vi "Scope_FPGA_v00.vi"(0 "Scope IPs":T3, 9 "Scope":T1, 11 "Lock Select":T4, 12 "Cavities Data":u64[](array[numeric]), 13 "XY HD ON":bool, 14 "Graph Data":u64[](array[numeric])) -> (1 "xy HD A":cluster{i16[], i16[]}(graph), 2 "xy HD B":cluster{i16[], i16[]}(graph), 3 "Scope OP Graph":cluster{dbl[], dbl[]}[](graph), 4 "Scope Cavities ON":bool, 6 "Scope Graph ON":bool, 8 "error":dbl[](array[numeric]), 10 "Scope Cavities":T2, 15 "Scope Graph":T2)   [LabVIEW 2010]
doc: "Creates an oscilliscope graph from the FIFO data, as well as packages data structures for FPGA_Cavities via the reference."
uses:
  Strict Type Defs/Lock Select.ctl
  Strict Type Defs/Lock or Hold.ctl
panel:
  out "Scope OPs (for saving)":cluster{dbl[], i16[], i16[], i16[], i16[]}
  in  "Scope":T2={"Trigger Direction"=enum."minus-plus", "Delay"=0, "Aquisition Rate (Ticks)"=20, "Offset"=0, "Channel"=0, "Channel Selector"={"Channel 1"=0, "Channel 2"=0, "Channel 3"=0, "Channel 4"=0}}
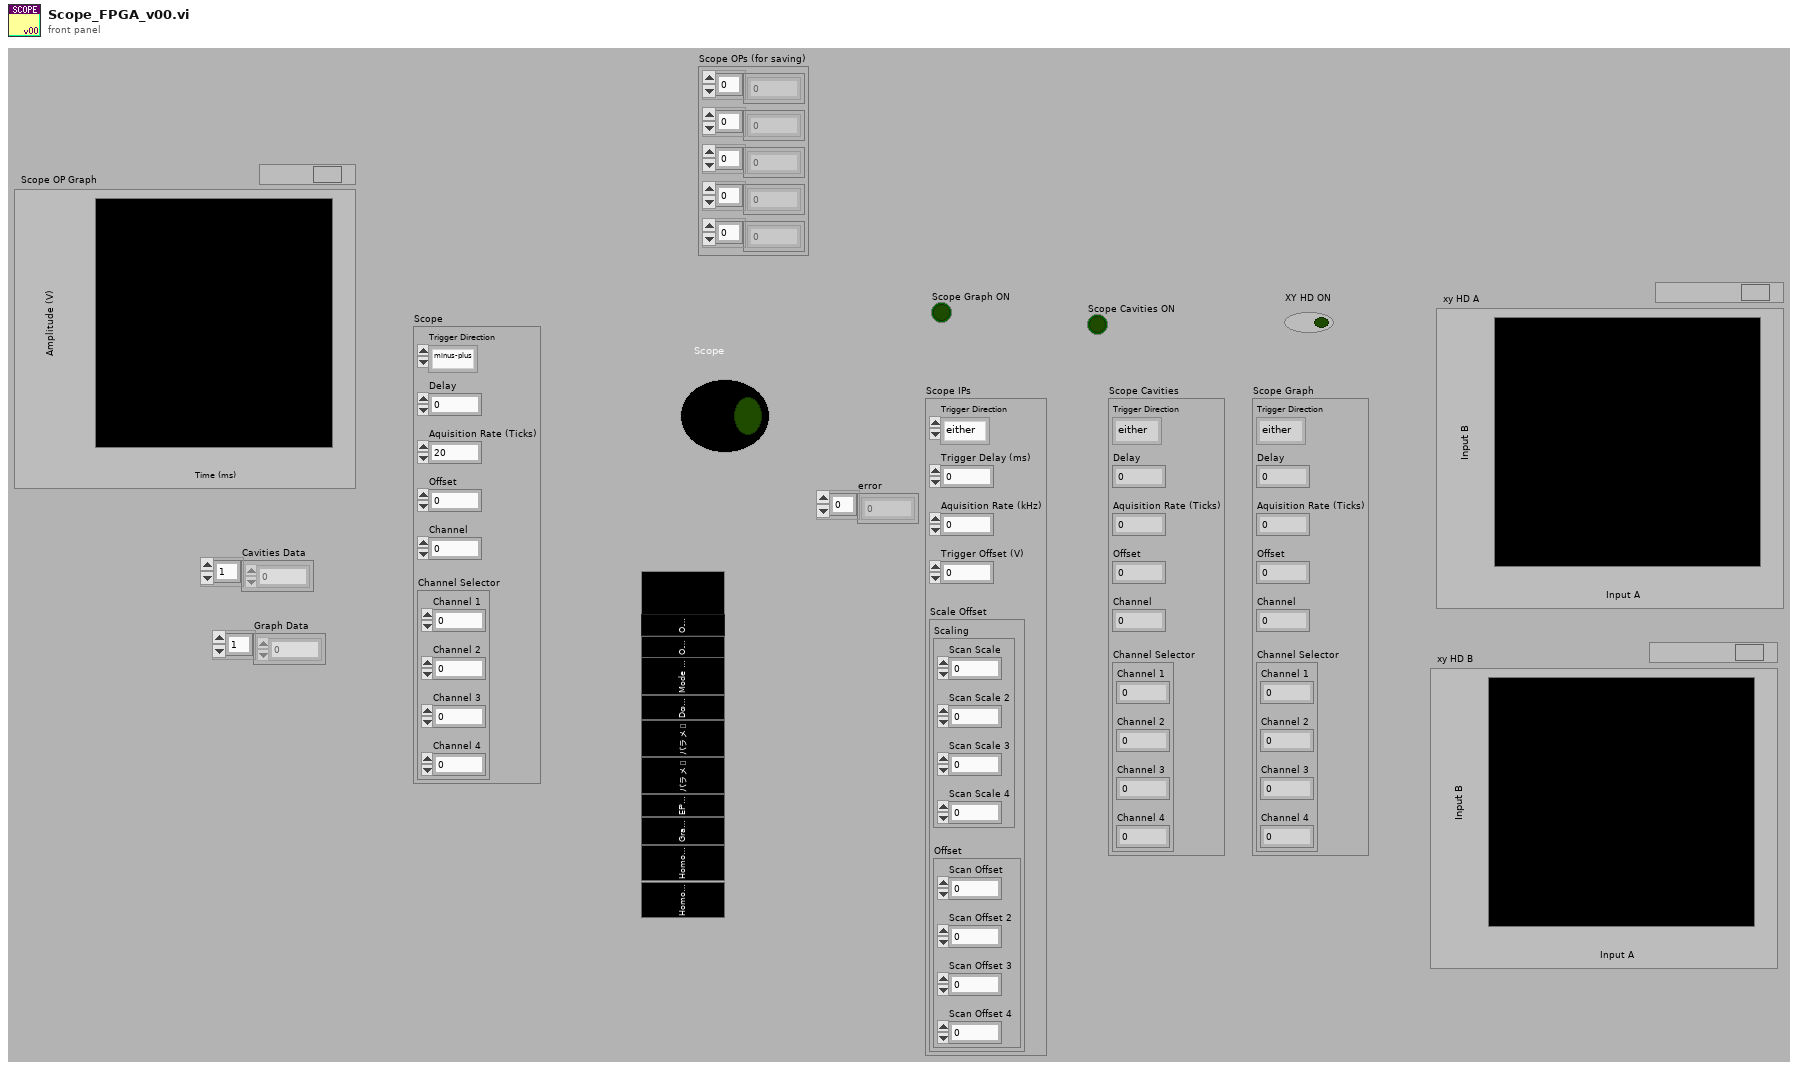
[diagram p1: front panel]
types:
  T1 = typedef "Lock or Hold.ctl" = bool
  T2 = cluster{"Trigger Direction":enum8{"either", "minus-plus", "plus-minus"}, "Delay":u32, "Aquisition Rate (Ticks)":u32, "Offset":i16, "Channel":i32, "Channel Selector":cluster{"Channel 1":i32, "Channel 2":i32, "Channel 3":i32, "Channel 4":i32}}
  T3 = cluster{"Trigger Direction":enum8{"either", "minus-plus", "plus-minus"}, "Trigger Delay (ms)":dbl, "Aquisition Rate (kHz)":dbl, "Trigger Offset (V)":dbl, "Scale Offset":cluster{"Scaling":cluster{"Scan Scale":i16, "Scan Scale 2":i16, "Scan Scale 3":i16, "Scan Scale 4":i16}, "Offset":cluster{"Scan Offset":i16, "Scan Offset 2":i16, "Scan Offset 3":i16, "Scan Offset 4":i16}}}
  T4 = typedef "Lock Select.ctl" = enum32{"OPO A", "OPO B", "Mode Cleaner", "Doubler", "パラメ OPO A", "パラメ OPO B", "EPR BS", "Graph BS", "Homodyne A", "Homodyne B"}
  T5 = cluster{"Channel 1":i32, "Channel 2":i32, "Channel 3":i32, "Channel 4":i32}
  T6 = cluster{"Scan Offset":i16, "Scan Offset 2":i16, "Scan Offset 3":i16, "Scan Offset 4":i16}
  T7 = cluster{"Scan Scale":i16, "Scan Scale 2":i16, "Scan Scale 3":i16, "Scan Scale 4":i16}
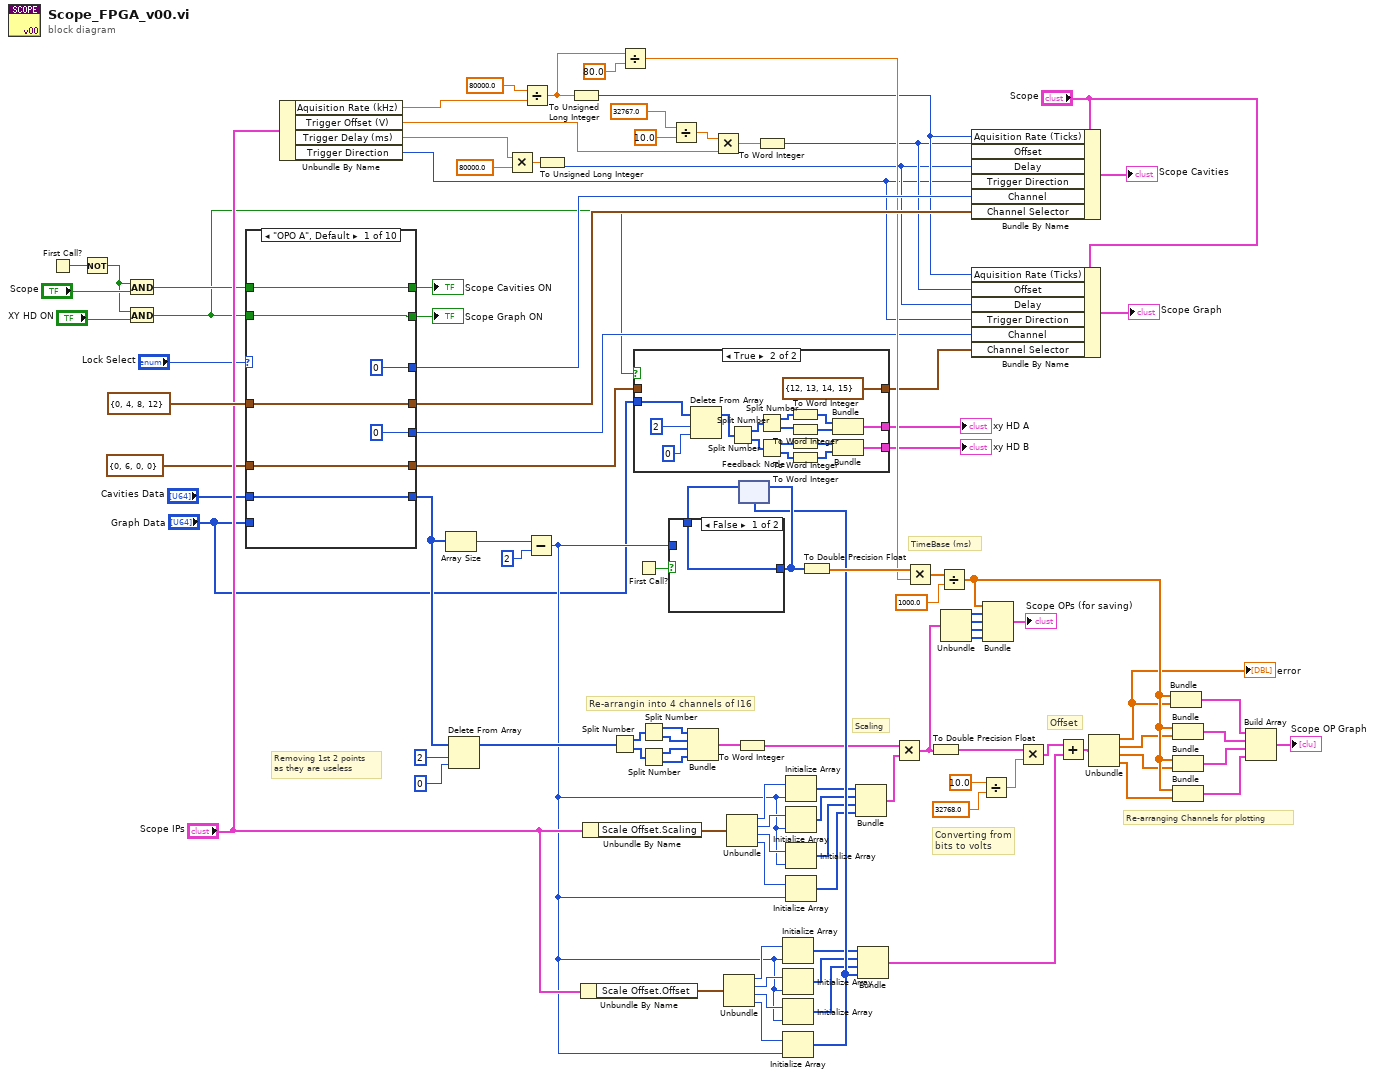
[diagram p0: block diagram]
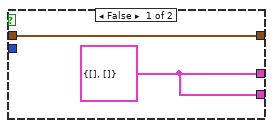
[diagram p2: hidden frame]
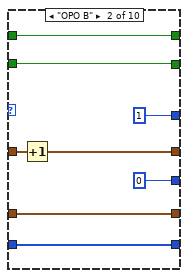
[diagram p4: hidden frame]
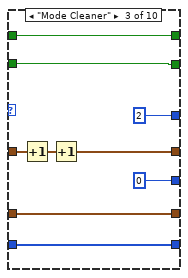
[diagram p5: hidden frame]
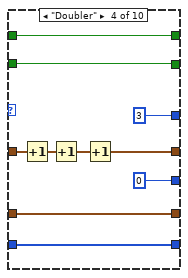
[diagram p6: hidden frame]
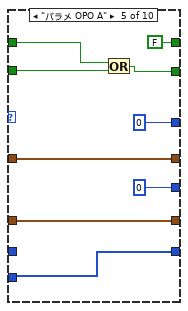
[diagram p7: hidden frame]
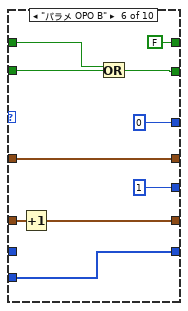
[diagram p8: hidden frame]
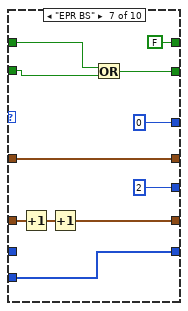
[diagram p9: hidden frame]
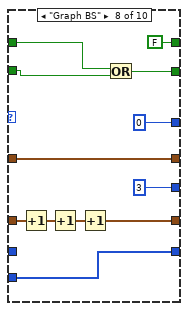
[diagram p10: hidden frame]
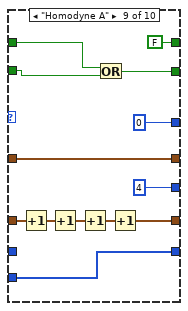
[diagram p11: hidden frame]
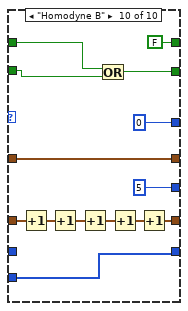
[diagram p12: hidden frame]
diagram:
  # "TimeBase (ms)"
  # "Re-arranging Channels for plotting"
  # "Re-arrangin into 4 channels of I16"
  # "Converting from\nbits to volts"
  # "Offset"
  # "Scaling"
  # "Removing 1st 2 points\nas they are useless"
  n1 = First Call?() -> (First Call?: T/F=w15:bool)
  n2 = Not(x=w15) -> (.not. x?=w7:bool)
  n3 = And(x=w7, y="Scope") -> (x .and. y?=w13:T1)
  n4 = And(x=w7, y="XY HD ON") -> (x .and. y?=w4:bool)
  n5 = case shown="\"OPO A\", Default" "Lock Select" {
    tunnel: T5 {"Channel 1"=0, "Channel 2"=4, "Channel 3"=8, "Channel 4"=12} ("Channel Selector") -> [w111 w116 w125 w135 w145 w155 w166 w178 w191 w205]
    tunnel: [w111 w115 w123 w131 w145 w155 w166 w178 w191 w205] -> w94
    tunnel: [0 1 2 3 0 0 0 0 0 0] -> w93
    tunnel: [w110 w119 w128 w138 w143 w152 w162 w173 w185 w198] -> w25
    tunnel: "Cavities Data" -> [w110 w119 w128 w138 _ _ _ _ _ _]
    tunnel: "Graph Data" -> [_ _ _ _ w143 w152 w162 w173 w185 w198]
    tunnel: [0 ("Channel") 0 ("Channel") 0 ("Channel") 0 ("Channel") 0 ("Channel") 1 ("Channel") 2 ("Channel") 3 ("Channel") 4 ("Channel") 5 ("Channel")] -> w17
    tunnel: T5 {"Channel 1"=0, "Channel 2"=6, "Channel 3"=0, "Channel 4"=0} ("Channel Selector") -> [w107 w114 w122 w133 w144 w154 w165 w177 w190 w204]
    tunnel: [w107 w114 w122 w133 w144 w153 w163 w174 w186 w199] -> w6
    tunnel: [w106 w113 w121 w130 T1 FALSE ("Scope") T1 FALSE ("Scope") T1 FALSE ("Scope") T1 FALSE ("Scope") T1 FALSE ("Scope") T1 FALSE ("Scope")] -> w14
    tunnel: w13 -> [w106 w113 w121 w130 w140 w148 w158 w169 w181 w194]
    tunnel: [w105 w112 w120 w129 w139 w149 w160 w171 w183 w196] -> w11
    tunnel: w4 -> [w105 w112 w120 w129 w141 w150 w159 w170 w182 w195]
    frame "OPO A", Default {
    }
    frame "OPO B" {
      n6 = Increment(x=w116) -> (x+1=w115:T5)
    }
    frame "Mode Cleaner" {
      n7 = Increment(x=w125) -> (x+1=w124:T5)
      n8 = Increment(x=w124) -> (x+1=w123:T5)
    }
    frame "Doubler" {
      n9 = Increment(x=w135) -> (x+1=w134:T5)
      n10 = Increment(x=w134) -> (x+1=w132:T5)
      n11 = Increment(x=w132) -> (x+1=w131:T5)
    }
    frame "パラメ OPO A" {
      n12 = Or(x=w140, y=w141) -> (x .or. y?=w139:T1)
    }
    frame "パラメ OPO B" {
      n13 = Increment(x=w154) -> (x+1=w153:T5)
      n14 = Or(x=w148, y=w150) -> (x .or. y?=w149:T1)
    }
    frame "EPR BS" {
      n15 = Increment(x=w165) -> (x+1=w164:T5)
      n16 = Increment(x=w164) -> (x+1=w163:T5)
      n17 = Or(x=w158, y=w159) -> (x .or. y?=w160:T1)
    }
    frame "Graph BS" {
      n18 = Increment(x=w177) -> (x+1=w176:T5)
      n19 = Increment(x=w176) -> (x+1=w175:T5)
      n20 = Increment(x=w175) -> (x+1=w174:T5)
      n21 = Or(x=w169, y=w170) -> (x .or. y?=w171:T1)
    }
    frame "Homodyne A" {
      n22 = Increment(x=w190) -> (x+1=w189:T5)
      n23 = Increment(x=w189) -> (x+1=w188:T5)
      n24 = Increment(x=w188) -> (x+1=w187:T5)
      n25 = Or(x=w181, y=w182) -> (x .or. y?=w183:T1)
      n26 = Increment(x=w187) -> (x+1=w186:T5)
    }
    frame "Homodyne B" {
      n27 = Increment(x=w204) -> (x+1=w203:T5)
      n28 = Increment(x=w203) -> (x+1=w202:T5)
      n29 = Increment(x=w202) -> (x+1=w201:T5)
      n30 = Or(x=w194, y=w195) -> (x .or. y?=w196:T1)
      n31 = Increment(x=w201) -> (x+1=w200:T5)
      n32 = Increment(x=w200) -> (x+1=w199:T5)
    }
  }
  "Scope Cavities ON" <- w14
  "Scope Graph ON" <- w11
  n33 = Unbundle By Name("Scope IPs") -> ("Aquisition Rate (kHz)"=w103:dbl, "Trigger Offset (V)"=w98:dbl, "Trigger Delay (ms)"=w96:dbl, "Trigger Direction"=w18:enum8{"either", "minus-plus", "plus-minus"})
  n34 = Array Size(array=w25) -> (size(s)=w87:i32)
  n35 = Delete From Array(array=w25, length=2, index=0) -> (array with subset deleted=w32:u64[])  [unwired: 1 out]
  n36 = Multiply(x=w96, y=80000.0) -> (x*y=w97:dbl)
  n37 = Divide(x=80000.0, y=w103) -> (x/y=w91:dbl)
  n38 = Subtract(x=w87, y=2) -> (x-y=w10:i32)
  n39 = To Unsigned Long Integer(number=w97) -> (unsigned 32bit integer=w19:u32)
  n40 = To Unsigned Long Integer(number=w91) -> (unsigned 32bit integer=w21:u32)
  n41 = Unbundle By Name("Scope IPs") -> ("Scale Offset.Offset"=w41:T6)
  n42 = Unbundle By Name("Scope IPs") -> ("Scale Offset.Scaling"=w57:T7)
  n43 = Split Number(x=w32) -> (hi(x)=w34:u32[], lo(x)=w33:u32[])
  n44 = Divide(x=w91, y=80.0) -> (x/y=w31:dbl)
  n45 = case shown="True" w4 {
    tunnel: w6 -> [w209 _]
    tunnel: [w209 T5 {"Channel 1"=12, "Channel 2"=13, "Channel 3"=14, "Channel 4"=15} ("Channel Selector")] -> w5
    tunnel: "Graph Data" -> [_ w211]
    tunnel: [w208 w215] -> w3
    tunnel: [w208 w214] -> w2
    frame False {
      w208 = cluster{i16[], i16[]} {[], []}
    }
    frame True {
      n46 = Delete From Array(array=w211, length=2, index=0) -> (array with subset deleted=w210:u64[])  [unwired: 1 out]
      n47 = Split Number(x=w210) -> (hi(x)=w224:u32[], lo(x)=w220:u32[])
      n48 = Split Number(x=w224) -> (hi(x)=w225:u16[], lo(x)=w223:u16[])
      n49 = Split Number(x=w220) -> (hi(x)=w219:u16[], lo(x)=w218:u16[])
      n50 = To Word Integer(number=w225) -> (16bit integer=w222:i16[])
      n51 = To Word Integer(number=w223) -> (16bit integer=w221:i16[])
      n52 = To Word Integer(number=w219) -> (16bit integer=w216:i16[])
      n53 = To Word Integer(number=w218) -> (16bit integer=w217:i16[])
      n54 = Bundle(w222, w221) -> (w215:cluster{i16[], i16[]})  [unwired: 1 in]
      n55 = Bundle(w216, w217) -> (w214:cluster{i16[], i16[]})  [unwired: 1 in]
    }
  }
  "xy HD A" <- w3
  "xy HD B" <- w2
  n56 = First Call?() -> (First Call?: T/F=w60:bool)
  n57 = Split Number(x=w34) -> (hi(x)=w83:u16[], lo(x)=w84:u16[])
  n58 = Split Number(x=w33) -> (hi(x)=w85:u16[], lo(x)=w86:u16[])
  n59 = Divide(x=32767.0, y=10.0) -> (x/y=w101:dbl)
  n60 = Bundle(w83, w84, w85, w86) -> (w58:cluster{u16[], u16[], u16[], u16[]})  [unwired: 1 out]
  n61 = Multiply(x=w101, y=w98) -> (x*y=w102:dbl)
  n62 = Unbundle(w41) -> ("Scan Offset"=w40:i16, "Scan Offset 2"=w44:i16, "Scan Offset 3"=w43:i16, "Scan Offset 4"=w42:i16)
  n63 = Unbundle(w57) -> ("Scan Scale"=w54:i16, "Scan Scale 2"=w53:i16, "Scan Scale 3"=w55:i16, "Scan Scale 4"=w56:i16)
  n64 = To Word Integer(number=w58) -> (16bit integer=w59:cluster{i16[], i16[], i16[], i16[]})
  n65 = To Word Integer(number=w102) -> (16bit integer=w20:i16)
  n66 = Initialize Array(w40, w10) -> (w45:i16[])
  n67 = Initialize Array(w44, w10) -> (w46:i16[])
  n68 = Initialize Array(w43, w10) -> (w47:i16[])
  n69 = Initialize Array(w42, w10) -> (w61:i16[])
  n70 = feedback #1(w61) -> (w62:i32[])
  n71 = case shown="False" w60 {
    tunnel: w10 -> [_ w229]
    tunnel: [w227 w228] -> w63
    tunnel: w62 -> [w227 _]
    frame False {
    }
    frame True {
      n72 = for {
        N: w229 -> [_]
        tunnel: [w230] -> w228 mode=indexing
        i -> [w230]
      }
    }
  }
  n73 = feedback-in #1(w63) -> ()
  n74 = Initialize Array(w54, w10) -> (w52:i16[])
  n75 = Initialize Array(w53, w10) -> (w51:i16[])
  n76 = Initialize Array(w55, w10) -> (w50:i16[])
  n77 = Initialize Array(w56, w10) -> (w49:i16[])
  n78 = To Double Precision Float(number=w63) -> (double precision float=w64:dbl[])
  n79 = Bundle(w52, w51, w50, w49) -> (w48:cluster{i16[], i16[], i16[], i16[]})  [unwired: 1 out]
  n80 = Bundle(w45, w46, w47, w61) -> (w39:cluster{i16[], i16[], i16[], i16[]})  [unwired: 1 out]
  n81 = Multiply(x=w59, y=w48) -> (x*y=w76:cluster{i16[], i16[], i16[], i16[]})
  n82 = Multiply(x=w64, y=w31) -> (x*y=w65:dbl[])
  n83 = To Double Precision Float(number=w76) -> (double precision float=w27:cluster{dbl[], dbl[], dbl[], dbl[]})
  n84 = Divide(x=w65, y=1000.0) -> (x/y=w81:dbl[])
  n85 = Unbundle(w76) -> (w77:i16[], w78:i16[], w79:i16[], w80:i16[])
  n86 = Bundle By Name(cluster="Scope", "Aquisition Rate (Ticks)"=w21, "Offset"=w20, "Delay"=w19, "Trigger Direction"=w18, "Channel"=w93, "Channel Selector"=w94) -> (→"Scope Cavities":T2)
  n87 = Bundle By Name(cluster="Scope", "Aquisition Rate (Ticks)"=w21, "Offset"=w20, "Delay"=w19, "Trigger Direction"=w18, "Channel"=w17, "Channel Selector"=w5) -> (→"Scope Graph":T2)
  n88 = Divide(x=10.0, y=32768.0) -> (x/y=w26:dbl)
  n89 = Bundle(w81, w77, w78, w79, w80) -> (→"Scope OPs (for saving)":cluster{dbl[], i16[], i16[], i16[], i16[]})  [unwired: 1 in]
  n90 = Multiply(x=w27, y=w26) -> (x*y=w37:cluster{dbl[], dbl[], dbl[], dbl[]})
  n91 = Add(x=w37, y=w39) -> (x+y=w38:cluster{dbl[], dbl[], dbl[], dbl[]})
  n92 = Unbundle(w38) -> (w67:dbl[], w68:dbl[], w69:dbl[], w70:dbl[])
  "error" <- w67
  n93 = Bundle(w81, w67) -> (w71:cluster{dbl[], dbl[]})  [unwired: 1 in]
  n94 = Bundle(w81, w68) -> (w72:cluster{dbl[], dbl[]})  [unwired: 1 in]
  n95 = Bundle(w81, w69) -> (w73:cluster{dbl[], dbl[]})  [unwired: 1 in]
  n96 = Bundle(w81, w70) -> (w74:cluster{dbl[], dbl[]})  [unwired: 1 in]
  n97 = Build Array(w71, w72, w73, w74) -> (→"Scope OP Graph":cluster{dbl[], dbl[]}[])
